vi "Write Astromech droid.lvclass.vi"(8 "error in (no error)":errorcluster, 10 "Astromech droid.lvclass":refnum<class "Astromech droid.lvclass">, 11 "X-wing in":refnum<class "X-wing.lvclass">) -> (0 "error out":errorcluster, 3 "X-wing out":refnum<class "X-wing.lvclass">)   [LabVIEW 2021, in "X-wing.lvclass"]
uses:
  X-wing.lvclass
  Astromech droid/Astromech droid.lvclass
  X-wing.lvclass/X-wing.ctl
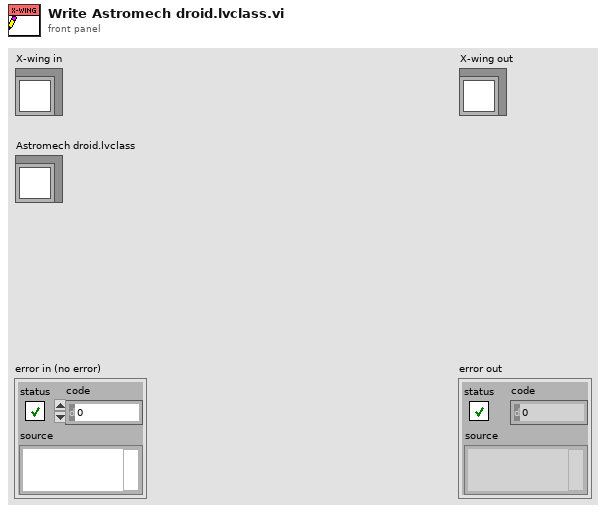
[diagram p1: front panel]
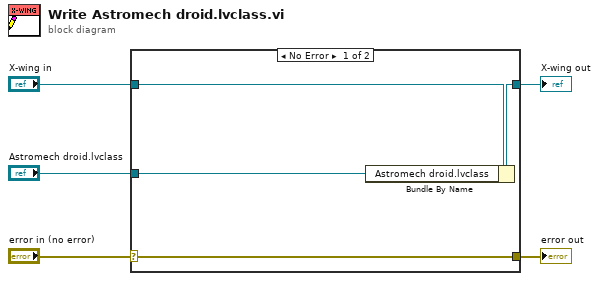
[diagram p0: block diagram]
diagram:
  n1 = case shown="No Error" "error in (no error)" {
    selector: "error in (no error)" -> [w9 w10]
    tunnel: [w9 w10] -> w4
    tunnel: [w7 w11] -> w2
    tunnel: "X-wing in" -> [w8 w11]
    tunnel: "Astromech droid.lvclass" -> [w6 _]
    frame No Error {
      n2 = Bundle By Name(cluster=w8, "Astromech droid.lvclass"=w6) -> (w7:refnum<class "X-wing.lvclass">)
    }
    frame Error {
    }
  }
  "error out" <- w4
  "X-wing out" <- w2
